vi "Set Cell Font.vi"(7 "Sheet Name":string, 8 "error in":errorcluster, 9 "Font":T1={"Bold"=enum."default", "Italic"=enum."default", "Underline"=enum."default", "TextColor"=0, "TextSize"=-1.0, "Name"=""}, 10 "Cell Address":string, 11 "SpreadsheetDoc in":refnum<k24>) -> (0 "error out":errorcluster, 3 "SpreadsheetDoc out":refnum<k24>)   [LabVIEW 2019, in "Open Xml.lvlib"]
uses:
  Open Xml.lvlib
  D:/git/Open-Xml-LabVIEW/Source/DocumentFormat.OpenXml.dll
  DocumentFormat.OpenXml.dll
  D:/git/Open-Xml-LabVIEW/Source/DocumentFormat.OpenXml.Framework.dll
  DocumentFormat.OpenXml.Framework.dll
  Font.ctl
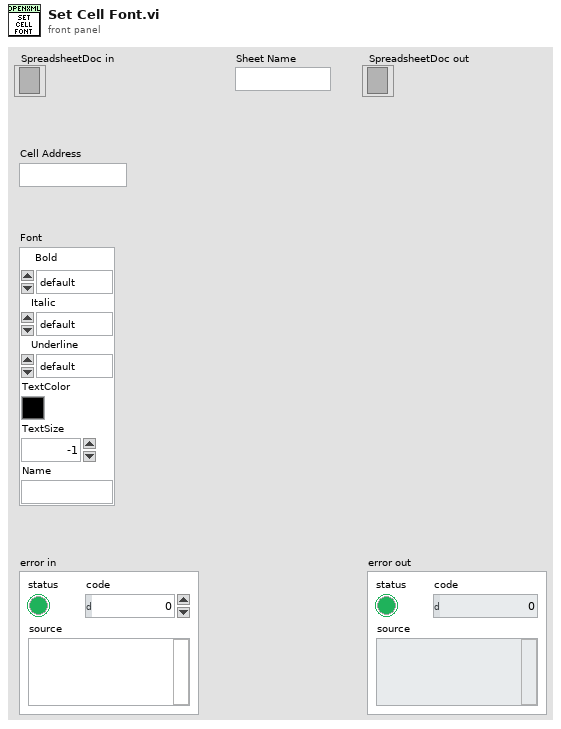
[diagram p1: front panel]
types:
  T1 = typedef "Open Xml.lvlib/Font.ctl" = cluster{"Bold":enum16{"bold", "regular", "default"}, "Italic":enum16{"italic", "regular", "default"}, "Underline":enum16{"single", "double", "singleAccounting", "doubleAccounting", "none", "default"}, "TextColor":u32, "TextSize":dbl, "Name":string}
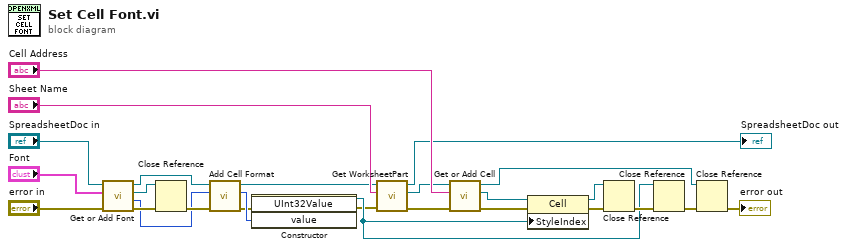
[diagram p0: block diagram]
diagram:
  n1 = call "Get or Add Font.vi"("error in"="error in", "Fonts"="Font", "SpreadsheetDoc in"="SpreadsheetDoc in") -> ("error out"=w22:errorcluster, "Font Id"=w7:i32, "Font"=w8:refnum<k24>, "SpreadsheetDoc out"=w11:refnum<k24>)  [unwired: 5 in]
  n2 = Close Reference(reference=w8, error in (no error)=w22) -> (error out=w9:errorcluster)
  n3 = call "Add Cell Format.vi"("error in"=w9, "Font Id"=w7, "SpreadsheetDoc in"=w11) -> ("error out"=w2:errorcluster, "Style Index"=w6:u32, "SpreadsheetDoc out"=w10:refnum<k24>)  [unwired: 6 in]
  n4 = constructor class="UInt32Value"(error in=w2, "value"=w6) -> (reference out=w5:refnum<k24>, error out=w1:errorcluster)  [unwired: 2 in, 2 out]
  n5 = call "Get WorksheetPart.vi"("error in"=w1, "Sheet Name"="Sheet Name", "SpreadsheetDocument in"=w10) -> ("error out"=w24:errorcluster, "WorksheetPart"=w17:refnum<k24>, "SpreadsheetDocument out"=→"SpreadsheetDoc out":refnum<k24>)  [unwired: 6 in]
  n6 = call "Get or Add Cell.vi"("error in"=w24, "Cell Address"="Cell Address", "Worksheetpart in"=w17) -> ("error out"=w3:errorcluster, "Cell"=w16:refnum<k24>, "WorksheetPart out"=w4:refnum<k24>)  [unwired: 6 in]
  n7 = property class="Cell"(reference=w16, error in=w3, "StyleIndex"=w5) -> (reference out=w13:refnum<k24>, error out=w19:errorcluster)
  n8 = Close Reference(reference=w13, error in (no error)=w19) -> (error out=w14:errorcluster)
  n9 = Close Reference(reference=w5, error in (no error)=w14) -> (error out=w12:errorcluster)
  n10 = Close Reference(reference=w4, error in (no error)=w12) -> (error out=→"error out":errorcluster)
